vi "write string.vi"() -> ()   [LabVIEW 2019]
uses:
  <vilib>/RTI DDS Toolkit/Types/RTI DDS Advanced Writer Configuration.ctl
  <vilib>/RTI DDS Toolkit/VIs/AdvancedCreateWriter_String.vi
  <vilib>/RTI DDS Toolkit/VIs/Write_String.vi
  <vilib>/RTI DDS Toolkit/Library/LVDDS_library.lvlib
panel:
  in  "type":string="%x %H-%M-%S "
  out "date/time string":string="2022-06-13 19-11-50 "
  out "decimal integer string":string="37"
  in  "stop":bool
  in  "Topic Name":string="rt/mystrtopic"
  in  "Domain Id":u32
  in  "Advanced Writer Configuration":T1={"typeName"="std_msgs::msg::dds_::String_", "keyName"="", "domainParticipantQoSProfile"="", "dataWriterQoSProfile"="", "forceArrayMapping?"=FALSE, "forceUnboundedString?"=FALSE}
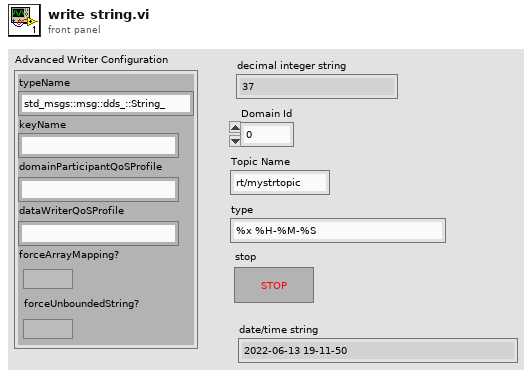
[diagram p1: front panel]
types:
  T1 = typedef "LVDDS_library.lvlib/RTI DDS Advanced Writer Configuration.ctl" = cluster{"typeName":string, "keyName":string, "domainParticipantQoSProfile":string, "dataWriterQoSProfile":string, "forceArrayMapping?":bool, "forceUnboundedString?":bool}
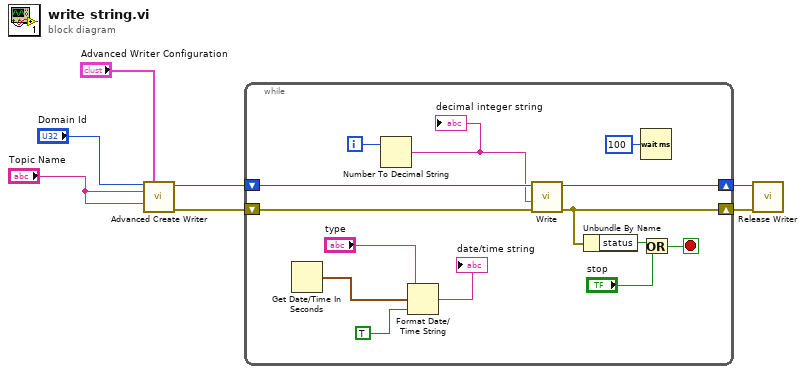
[diagram p0: block diagram]
diagram:
  n1 = call-poly <vilib>:"Advanced Create Writer.vi"("Domain Id"="Domain Id", "Advanced Writer Configuration"="Advanced Writer Configuration", "Topic Name"="Topic Name", "Data Type"="Topic Name") -> ("DDS Object Ref"=w4:u64, "error out"=w7:errorcluster)  [unwired: 10 in]
  n2 = while {
    shift-right: [w17] -> w6
    shift-left: w7 -> [w21]
    shift-right: [w20] -> w5
    shift-left: w4 -> [w19]
    i -> [w18]
    stop <- w15 stop-if-true
    n3 = Get Date/Time In Seconds() -> (seconds since 1Jan1904=w9:timestamp)
    n4 = Number To Decimal String(number=w18) -> (decimal integer string=w12:string)  [unwired: 1 in]
    "decimal integer string" <- w12
    n5 = Format Date/Time String(time format string (%c)="type", seconds (now)=w9, UTC format=TRUE) -> (date/time string=→"date/time string":string)
    n6 = call-poly <vilib>:"Write.vi"("error in (no error)"=w21, "Data"=w12, "DDS Object Ref in"=w19) -> ("error out"=w17:errorcluster, "DDS Object Ref out"=w20:u64)  [unwired: 7 in]
    n7 = Unbundle By Name(w17) -> ("status"=w16:bool)
    n8 = Wait (ms)(milliseconds to wait=u32 100) -> ()  [unwired: 1 out]
    n9 = Or(x=w16, y="stop") -> (x .or. y?=w15:bool)
  }
  n10 = call <vilib>:"Release Writer.vi"("error in (no error)"=w6, "DDS Object Ref"=w5) -> ()  [unwired: 9 in, 1 out]
